vi "niSwitch Wait For Debounce Wrapper.vi"(8 "error in":errorcluster, 10 "maximum time (5000 ms)":i32=5000, 11 "session factory in":refnum<class "Session Factory.lvclass">) -> (0 "error out":errorcluster, 3 "session factory out":refnum<class "Session Factory.lvclass">)   [LabVIEW 2021, in "Session Management niSwitch.lvlib" / "Session Factory.lvclass"]
doc: "Pauses until all created paths have settled. Call this VI before the niSwitch Get Relay Count VI to ensure an accurate relay count."
uses:
  Session Factory.lvclass
  NI Switch_client/RPC Messages/niswitch_grpc_WaitForDebounceRequest.ctl
  NI Switch_client/RPC Messages/nidevice_grpc_Session.ctl
  NI Switch_client/RPC Messages/nidevice_grpc_Session_session/nidevice_grpc_Session_session.lvclass
  Session Factory.lvclass/Session Factory.ctl
  NI Switch_client/NI Switch_client.lvlib
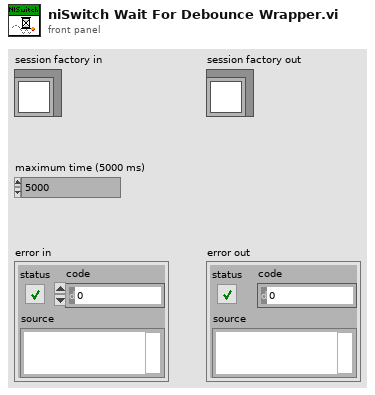
[diagram p1: front panel]
types:
  T1 = typedef "NI Switch_client.lvlib/niswitch_grpc_WaitForDebounceRequest.ctl" = cluster{"vi":T2, "maximum_time_ms":i32}
  T2 = typedef "NI Switch_client.lvlib/nidevice_grpc_Session.ctl" = cluster{"nidevice_grpc_Session_session":refnum<class "nidevice_grpc_Session_session.lvclass">}
  T3 = typedef "grpc-lvsupport-release.lvlib/grpcId.ctl" = u64
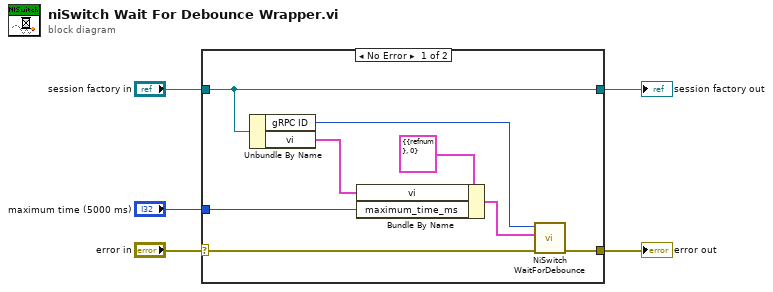
[diagram p0: block diagram]
diagram:
  n1 = case shown="No Error" "error in" {
    selector: "error in" -> [w7 w14]
    tunnel: [w12 w15] -> w4
    tunnel: "session factory in" -> [w12 w15]
    tunnel: [w11 w14] -> w3
    tunnel: "maximum time (5000 ms)" -> [w9 _]
    frame No Error {
      n2 = Unbundle By Name(w12) -> ("gRPC ID"=w6:T3, "vi"=w13:T2)
      n3 = Bundle By Name(cluster=T1 {"vi"={"nidevice_grpc_Session_session"=refnum}, "maximum_time_ms"=0} ("Request Data"), "vi"=w13, "maximum_time_ms"=w9) -> (w10:T1)
      n4 = call "NiSwitch WaitForDebounce.vi"("error in"=w7, "Request Data"=w10, "gRPC ID"=w6) -> ("error out"=w11:errorcluster)  [unwired: 6 in, 2 out]
    }
    frame Error {
    }
  }
  "error out" <- w3
  "session factory out" <- w4
